vi "FIB profile.vi"(1 "ActiveX Container":refnum<k7>(container), 4 "Capella HV Data Output":T2 {"Column Vac (Torr)" format="%.2e"; "Gun Vac (Torr)" format="%.2e"; "Lens2 Actual (V)" format="%.1f"; "Lens1 Actual (V)" format="%.1f"; "Emission Actual (uA)" format="%.3f"; "Extrator Actual (V)" format="%.1f"; "Tip Lifetime (uAhr)" format="%.2f"; "Lens2 Target (V)" format="%.1f"; "Lens1 Target (V)" format="%.1f"; "SuppI (uA)" format="%.3f"; "Suppressor (V)" format="%.1f"; "Emission Target (uA)" format="%.3f"; "Extrator Target (V)" format="%.1f"; "Accelerator Actual (V)" format="%.1f"; "Accelerator Target (V)" format="%.1f"; "Filament (A)" format="%.2f"}, 5 "HV Data Output":T3 {"Tip Lifetime (hr)" format="%.2f"; "Lens2I (uA)" format="%.3f"; "Lens2 (V)" format="%.1f"; "Lens1I (uA)" format="%.3f"; "Lens1 (V)" format="%.1f"; "SuppI (uA)" format="%.3f"; "Suppressor (V)" format="%.1f"; "Emission (uA)" format="%.3f"; "Extrator (V)" format="%.1f"; "AccI (uA)" format="%.3f"; "Acclerator (V)" format="%.1f"; "Filament (A)" format="%.2f"}, 6 "Parameter Names":string[](array[string])=["Faraday Cup Current", "Specimen Current", "Beam Dump 1 Current", "Beam Dump 2 Current"], 7 "Active logging channels":string="Log/ai0:3", 8 "Scan Para":T5={"X resolution"=500, "Z resolution"=500, "X center"=0.0, "Z center"=0.0, "X size (V)"=10.0, "Z size (V)"=10.0, "Frame line rampdown ratio"=-0.1, "Scan rate (Hz)"=2000000, "Oversampling"=2} {"Frame line rampdown ratio" min=-1.0 max=1.0 step=0.05 format="%.2g"; "Scan rate (Hz)" max=4000000 format="%#.6p"}, 9 "Milling para":T1={"X resolution"=4096, "Z resolution"=125001, "X offset (um)"=0.0, "Z offset (um)"=0.0, "X center (um)"=0.0, "Z center (um)"=0.0, "X size (um)"=250.0, "Z size (um)"=250.0, "UL-Ang"=90.0, "UR-Ang"=90.0, "Line milling time (s)"=5.0, "Z-step (nm)"=2.0, "Lines auto pause"=1, "Auto pause"=FALSE, "Mill from Bottom"=FALSE, "FIB FOV (um)"=500.0, "Auto Profile"=FALSE, "Mill start from Last"=FALSE, "FIB PID on"=FALSE, "FIB PID reset"=TRUE, "FIB PID measured"=0, "FIB PID target"=0.0, "FIB PID target slope"=0.0, "FIB PID P"=0.001, "FIB PID I"=0.01, "FIB PID D"=0.0, "Emission (uA)"=1.36, "Suppressor (V)"=50.0, "Auto reheat"=FALSE} caption="Milling Parameters" {"Suppressor (V)" step=0.1 format="%.1g"; "Emission (uA)" step=0.1 format="%.2g"; "FIB PID measured" items=["Spec.", "B.D. 1", "B.D. 2", "Mill", "Spec. +"]; "FIB PID target slope" min=-1 max=1 step=0.1; "UR-Ang" format="%.2f"; "UL-Ang" format="%.2f"; "Z offset (um)" step=0.02 format="%.3g"; "X offset (um)" step=1 format="%.3g"; "FIB FOV (um)" format="%.3g"; "Line milling time (s)" format="%.1f"; "Z center (um)" format="%#.3g"; "X center (um)" format="%#.3g"}, 10 "Options":T6 {"Scan mode" items=["Raster", "Serpentine"]; "Det" items=["Detector A", "Detector B"]}, 11 "HW Config":T7={"FIB X coil"="FIB/ao0", "FIB Y coil"="FIB/ao1", "Beam blank"="FIB/port0/line0", "Ext Scan"="FIB/port0/line1", "Detector"="FIB/ai1", "Shutter Drive"="PXI1Slot2/ao0"}) -> (0 "error out":errorcluster, 2 "Measurements":dbl[][](graph), 3 "Info & Status":T4={"Actual scan rate"=2000000.0, "X resolution with rampdown"=552, "Actual sample rate"=4000000.0, "Fetch backlog"=664878.0, "Total scan points"=276000, "Frame rate (/s)"=7} {"Fetch backlog" format="%#_6p"; "Actual sample rate" format="%#_6p"; "Actual scan rate" format="%#_4p"})   [LabVIEW 2018]
uses:
  <vilib>/DAQmx/write.llb/DAQmx Write (Digital Wfm 1Chan NSamp).vi
  <vilib>/DAQmx/write.llb/DAQmx Write (Analog 2D DBL NChan NSamp).vi
  <vilib>/DAQmx/read.llb/DAQmx Read (Analog 2D DBL NChan NSamp).vi
  <vilib>/DAQmx/create/channels.llb/DAQmx Create Channel (AI-Voltage-Basic).vi
  <vilib>/Waveform/DWDTOps.llb/DWDT Invert Digital.vi
  <vilib>/DAQmx/create/channels.llb/DAQmx Create Channel (AO-Voltage-Basic).vi
  <vilib>/DAQmx/create/channels.llb/DAQmx Create Channel (DO-Digital Output).vi
  <vilib>/Waveform/DWDTOps.llb/Digital Pattern Generator (Single Value).vi
  <vilib>/Waveform/DWDTOps.llb/DWDT Replace Subset.vi
  <vilib>/DAQmx/configure/timing.llb/DAQmx Timing (Sample Clock).vi
  <vilib>/DAQmx/create/channels.llb/DAQmx Create Channel (CO-Pulse Generation-Frequency).vi
  <vilib>/DAQmx/configure/trigger.llb/DAQmx Start Trigger (Digital Edge).vi
  <vilib>/Waveform/DWDTOps.llb/DWDT Uncompress Digital.vi
  <vilib>/DAQmx/miscellaneous.llb/DAQmx Fill In Error Info.vi
  <vilib>/Utility/file.llb/Write To Spreadsheet File (string).vi
  <resource>/objmgr/daqmx.rc
panel:
  out "Blanking":digitalwaveform(graph)
  in  "COM port":refnum<visa-resource-name>="COM1"
  out "Mill from Bottom":bool
  out "Y scan pattern":dbl[](array[numeric])
  out "AI SampleClk.MaxRate":dbl
  in  "Machine Type":u8(ring) items=["Feiss", "NVision", "Jeiss"]
  out "Ext scan":tag
  out "FIB Y coil":tag="PXI1Slot7/ao1"
  out "FIB X coil":tag="PXI1Slot7/ao0"
  in  "Beam blanked":bool
  out "Beam blank":tag="PXI1Slot7/port0/line0"
  out "Oversampling":u16=2
  out "Frame line rampdown ratio":dbl=0.1
  out "Y end":dbl=1.0
  out "X end":dbl=1.0
  out "Y start":dbl=-1.0
  out "X start":dbl=-1.0
  out "Y resolution":u32=500
  out "X resolution":u32=500
  out "Flip z":bool
  out "Flip x":bool
  out "Scan mode":u16
  in  "stop":bool=TRUE
  # "Direction"
  # "Start\nfrom"
  # "<"
  # "Flip"
  # "Scan coils"
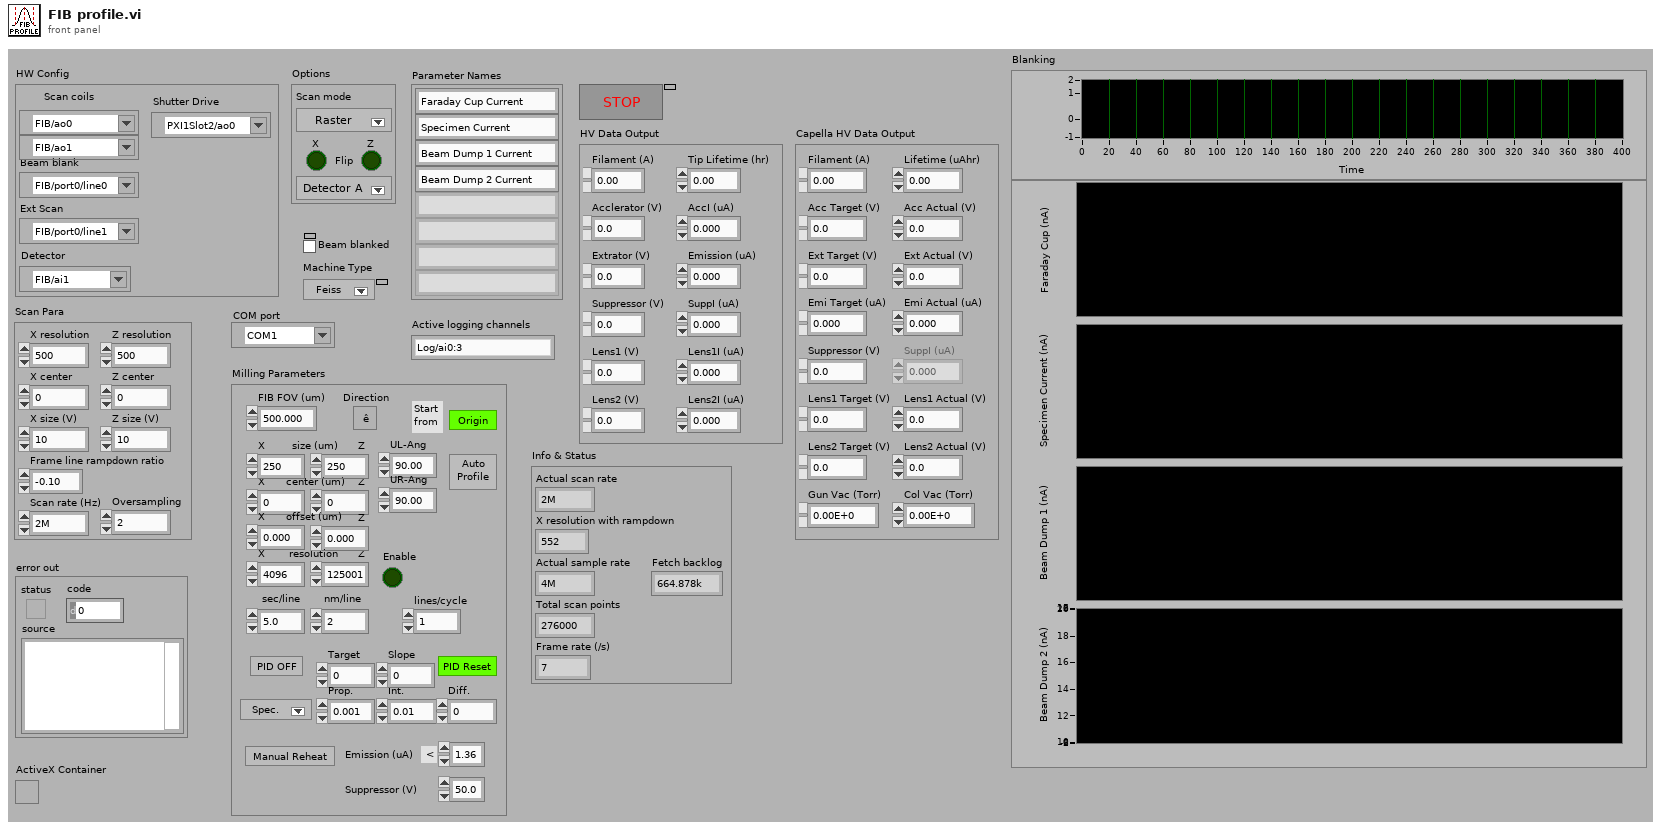
[diagram p1: front panel]
types:
  T1 = cluster{"X resolution":u32, "Z resolution":u32, "X offset (um)":sgl, "Z offset (um)":sgl, "X center (um)":sgl, "Z center (um)":sgl, "X size (um)":sgl, "Z size (um)":sgl, "UL-Ang":sgl, "UR-Ang":sgl, "Line milling time (s)":sgl, "Z-step (nm)":dbl, "Lines auto pause":u16, "Auto pause":bool, "Mill from Bottom":bool, "FIB FOV (um)":sgl, "Auto Profile":bool, "Mill start from Last":bool, "FIB PID on":bool, "FIB PID reset":bool, "FIB PID measured":u8, "FIB PID target":sgl, "FIB PID target slope":sgl, "FIB PID P":sgl, "FIB PID I":sgl, "FIB PID D":sgl, "Emission (uA)":dbl, "Suppressor (V)":sgl, "Auto reheat":bool}
  T2 = cluster{"Filament (A)":sgl, "Accelerator Target (V)":sgl, "Accelerator Actual (V)":sgl, "Extrator Target (V)":sgl, "Extrator Actual (V)":sgl, "Emission Target (uA)":sgl, "Emission Actual (uA)":sgl, "Suppressor (V)":sgl, "SuppI (uA)":sgl, "Lens1 Target (V)":sgl, "Lens1 Actual (V)":sgl, "Lens2 Target (V)":sgl, "Lens2 Actual (V)":sgl, "Gun Vac (Torr)":sgl, "Column Vac (Torr)":sgl, "Tip Lifetime (uAhr)":sgl}
  T3 = cluster{"Filament (A)":sgl, "Acclerator (V)":sgl, "AccI (uA)":sgl, "Extrator (V)":sgl, "Emission (uA)":sgl, "Suppressor (V)":sgl, "SuppI (uA)":sgl, "Lens1 (V)":sgl, "Lens1I (uA)":sgl, "Lens2 (V)":sgl, "Lens2I (uA)":sgl, "Tip Lifetime (hr)":sgl}
  T4 = cluster{"Actual scan rate":dbl, "X resolution with rampdown":i32, "Actual sample rate":dbl, "Fetch backlog":dbl, "Total scan points":i32, "Frame rate (/s)":u32}
  T5 = cluster{"X resolution":u32, "Z resolution":u32, "X center":dbl, "Z center":dbl, "X size (V)":dbl, "Z size (V)":dbl, "Frame line rampdown ratio":dbl, "Scan rate (Hz)":u32, "Oversampling":u16}
  T6 = cluster{"Scan mode":u16, "Flip x":bool, "Flip z":bool, "Det":u16}
  T7 = cluster{"FIB X coil":tag, "FIB Y coil":tag, "Beam blank":tag, "Ext Scan":tag, "Detector":tag, "Shutter Drive":tag}
  T8 = enum16{"SEM", "FIB", "Milling", "SEM + FIB", "Mill + SEM", "SEM Drift Correction", "FIB Drift Correction", "No Beam", "External", "External + SEM"}
  T9 = enum16{"SEM", "FIB", "Mill", "SEM + FIB", "Mill + SEM", "Drift SEM", "Drift FIB", "None", "Ext", "Ext + SEM"}
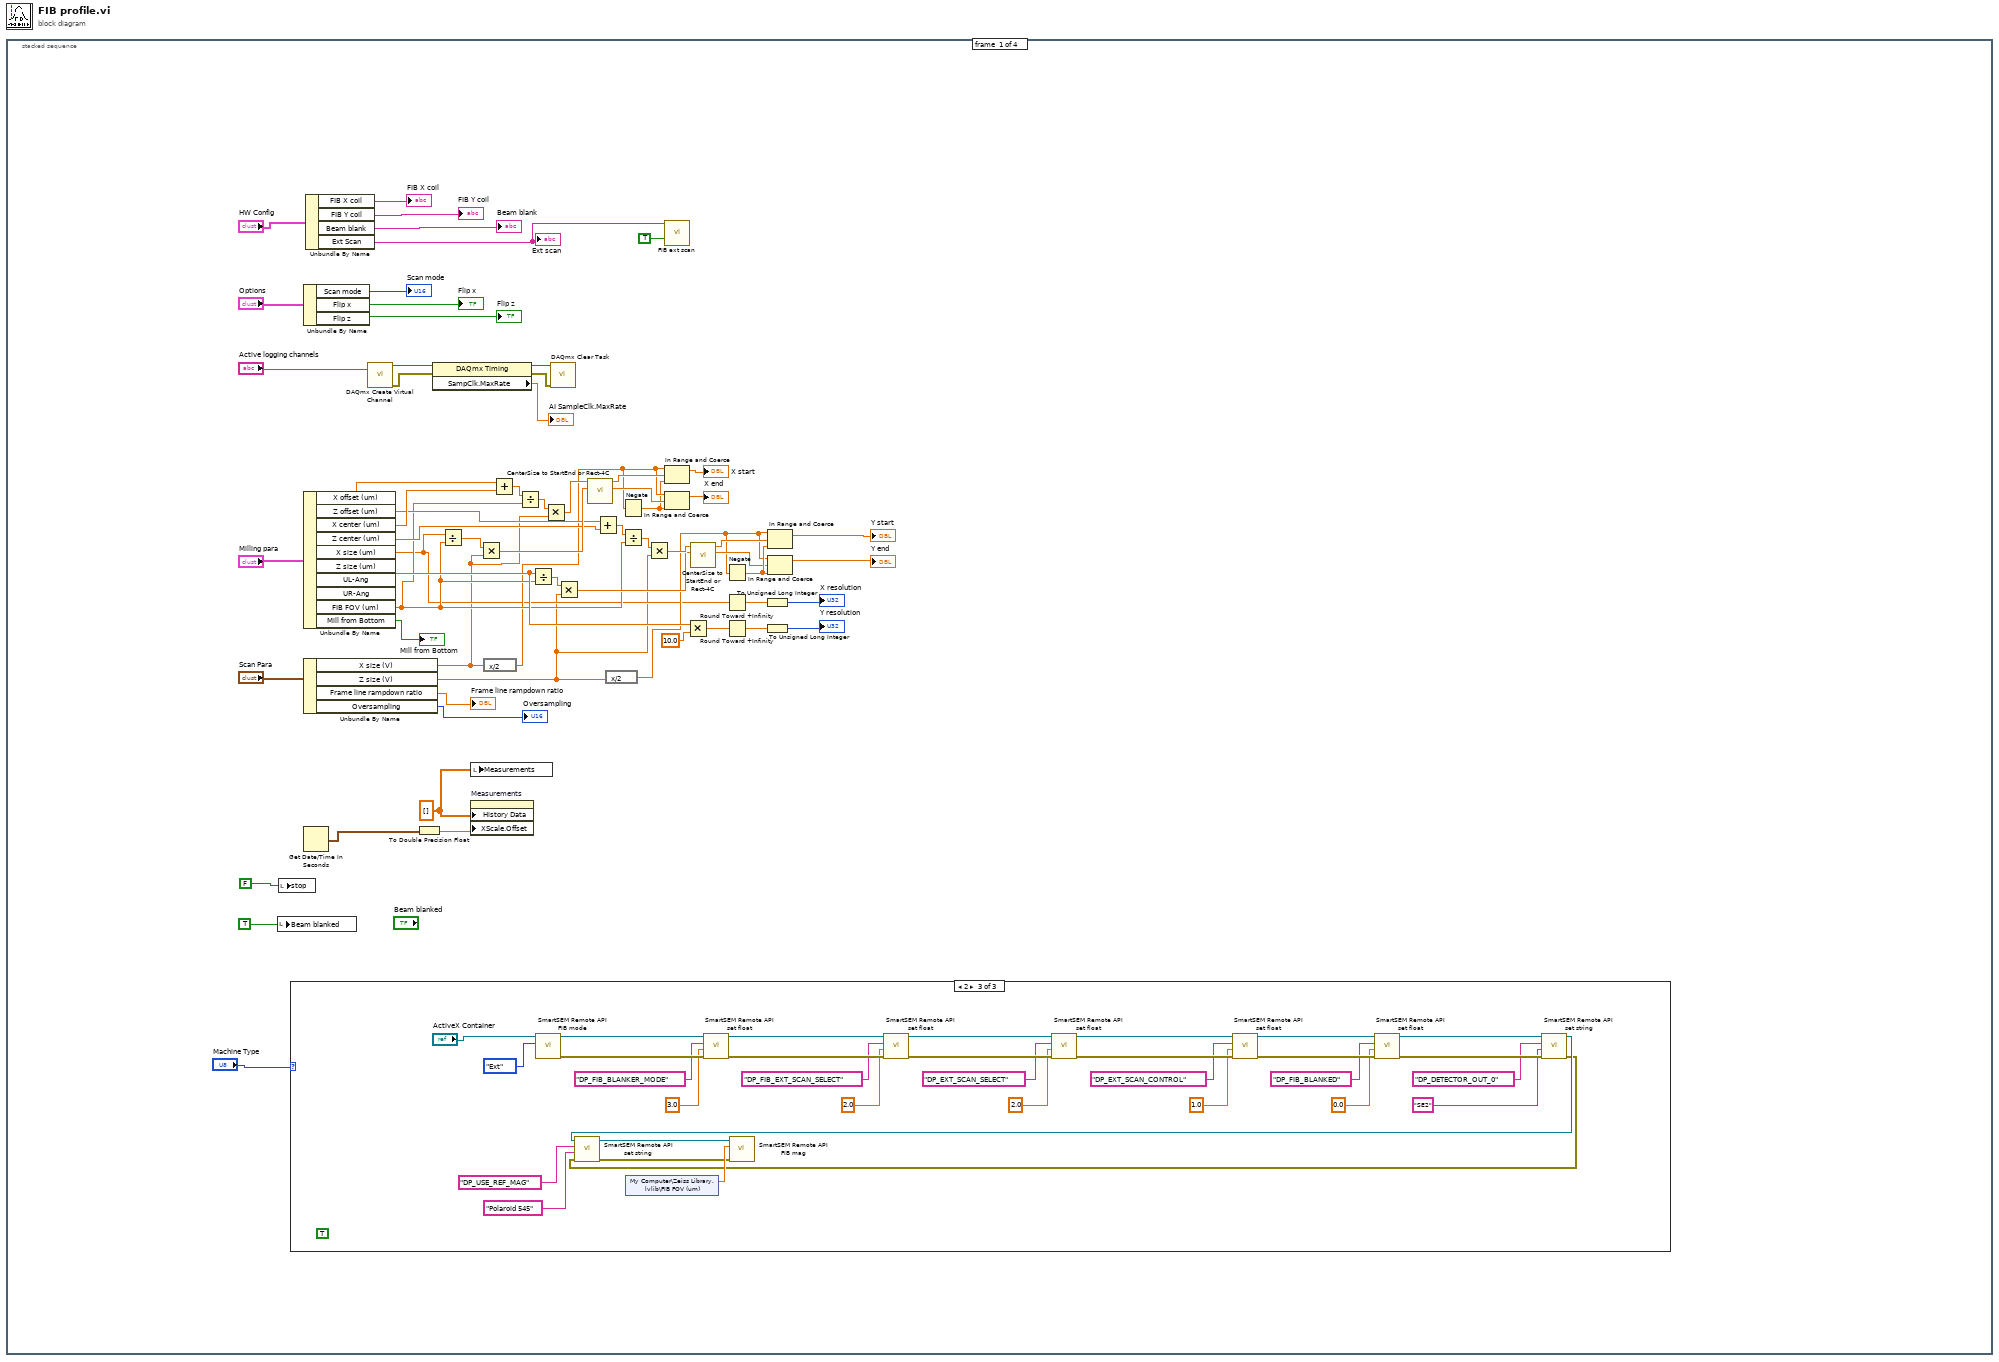
[diagram p0: block diagram]
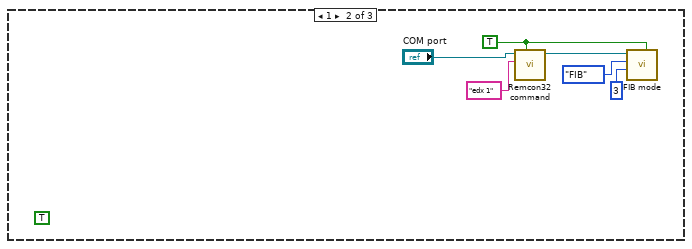
[diagram p3: hidden frame]
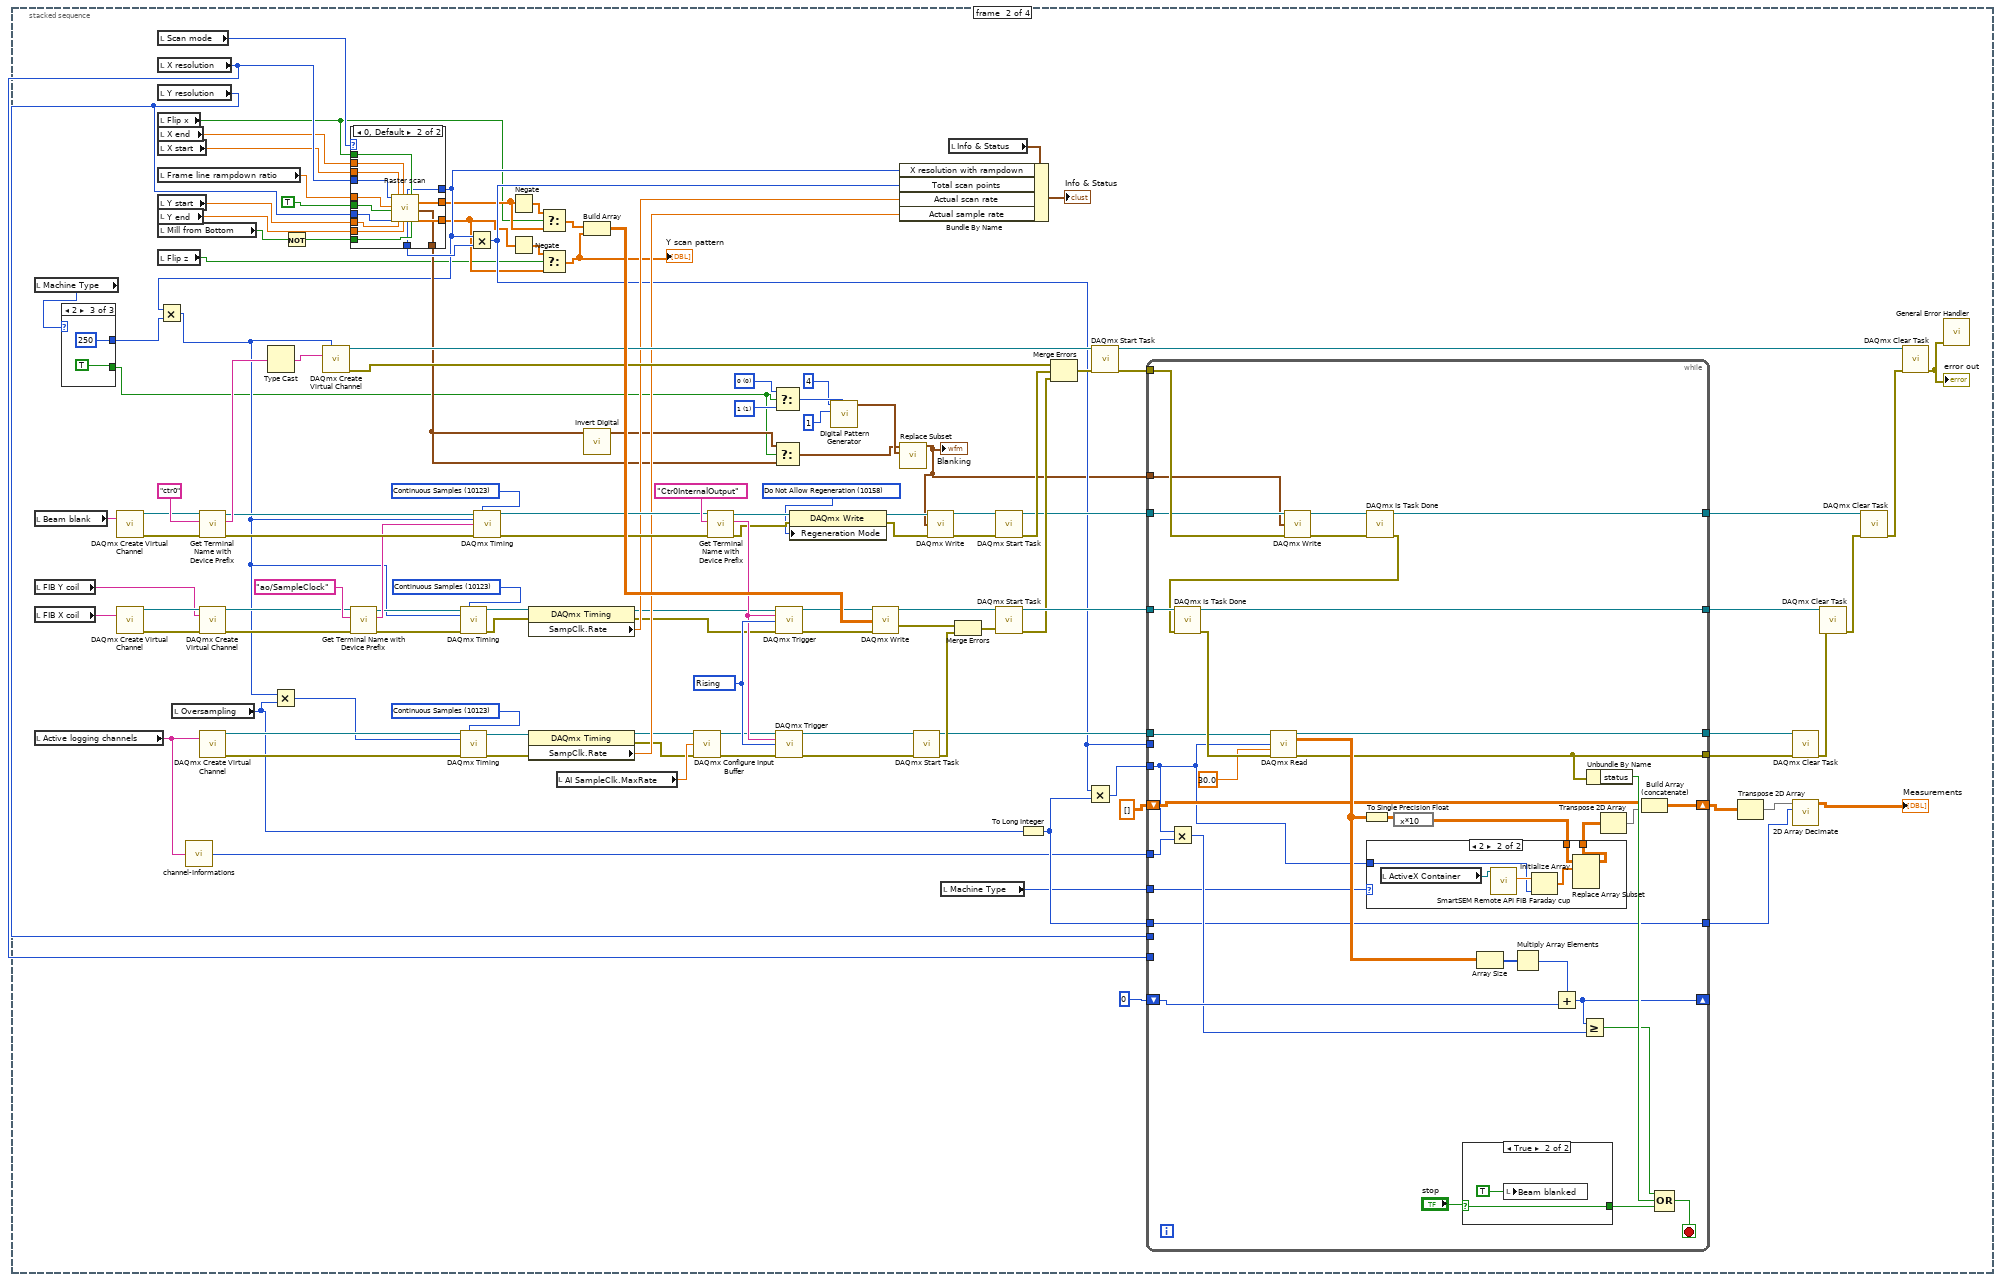
[diagram p4: hidden frame]
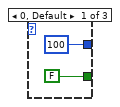
[diagram p5: hidden frame]
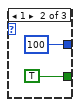
[diagram p6: hidden frame]
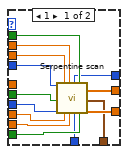
[diagram p7: hidden frame]
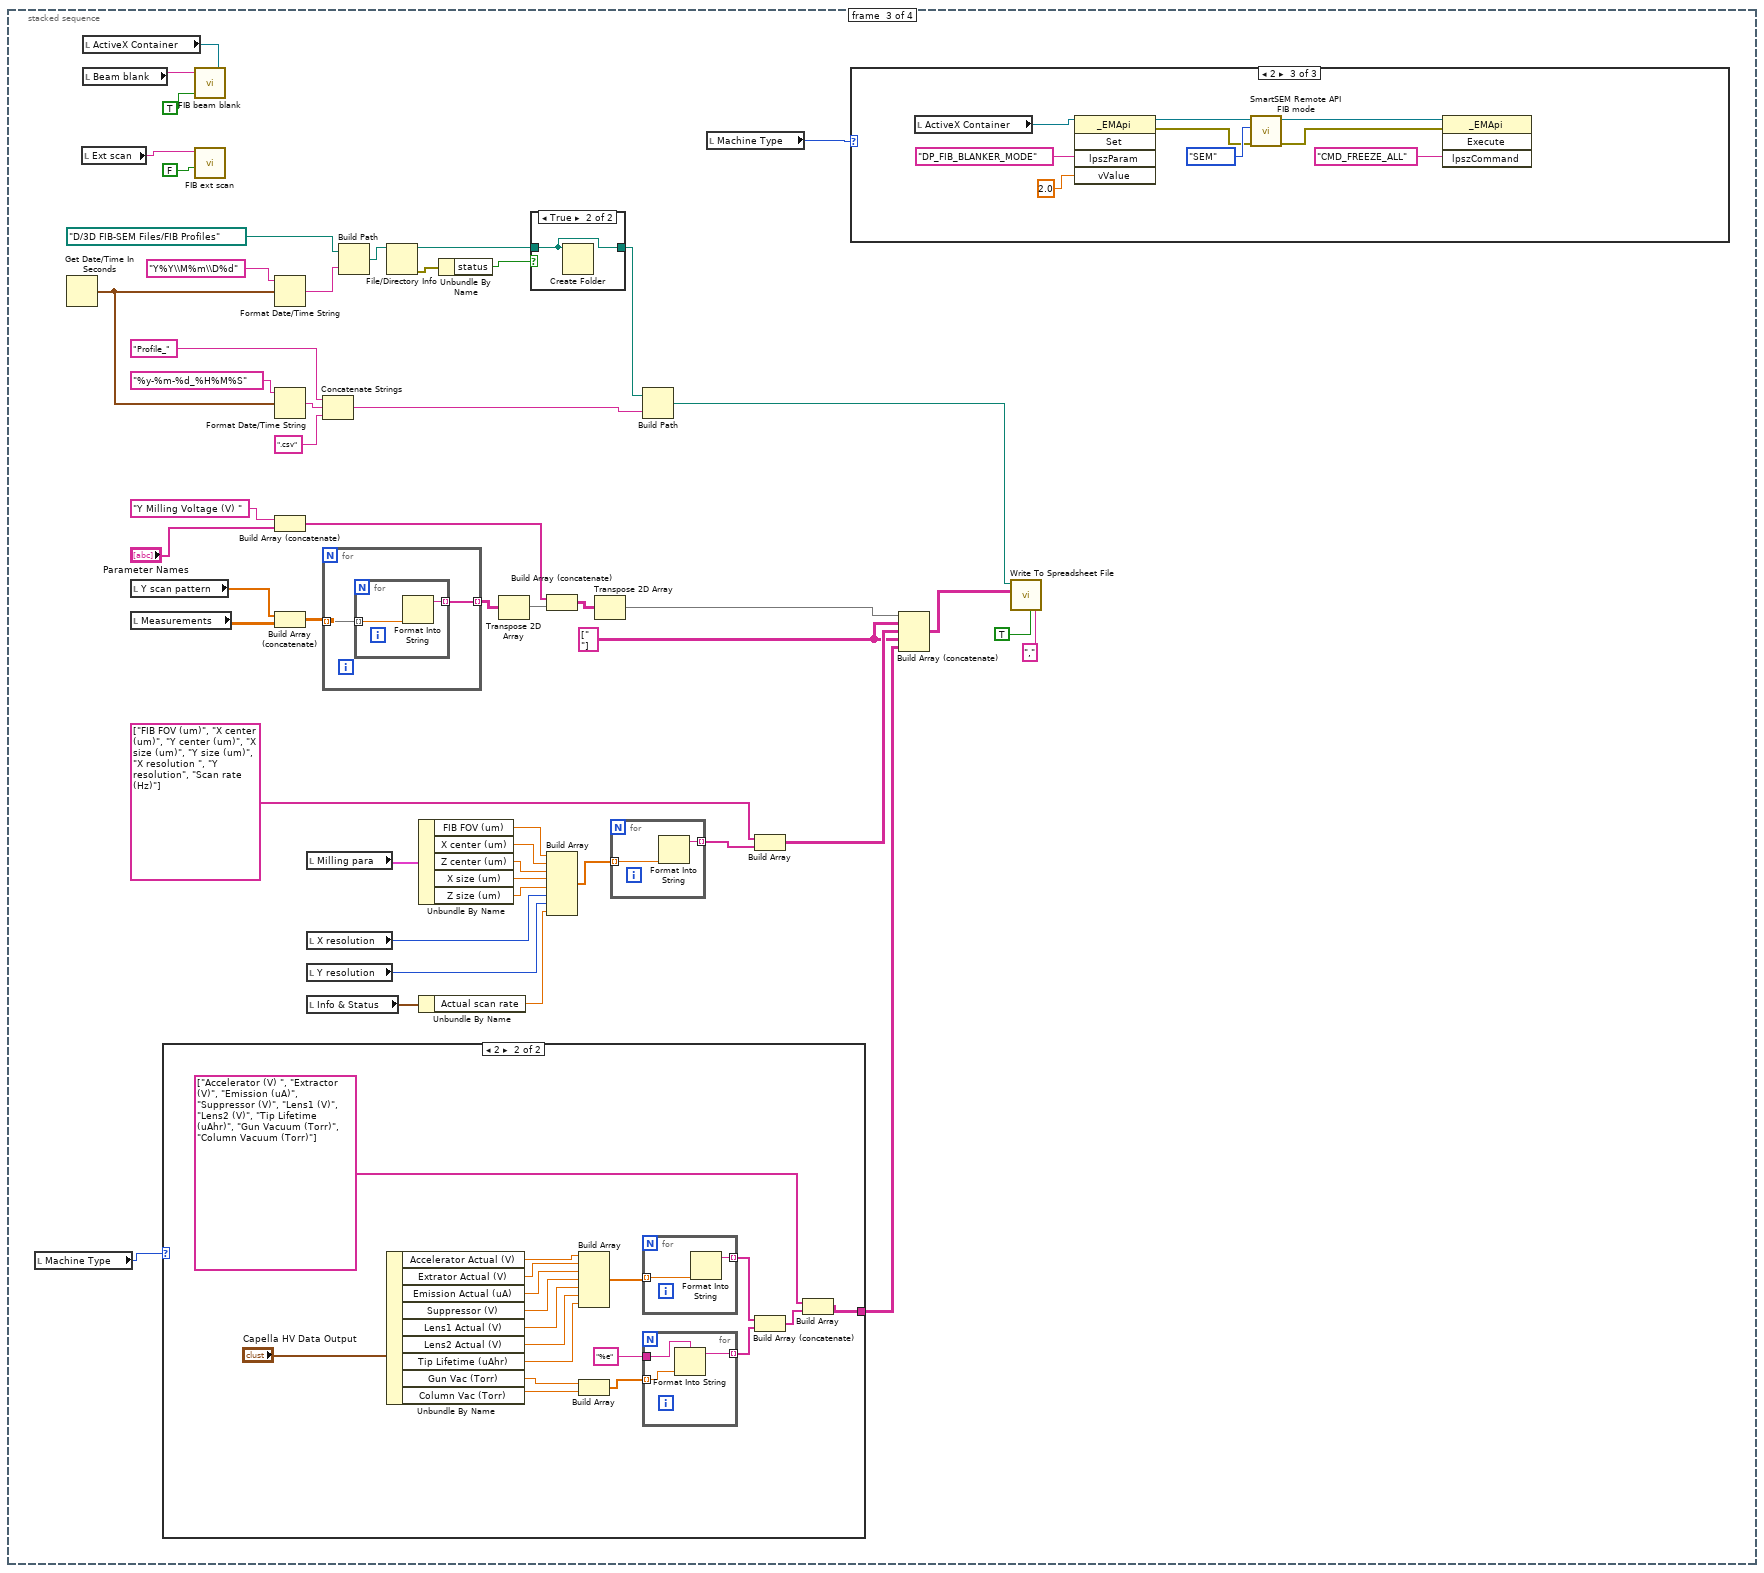
[diagram p10: hidden frame]
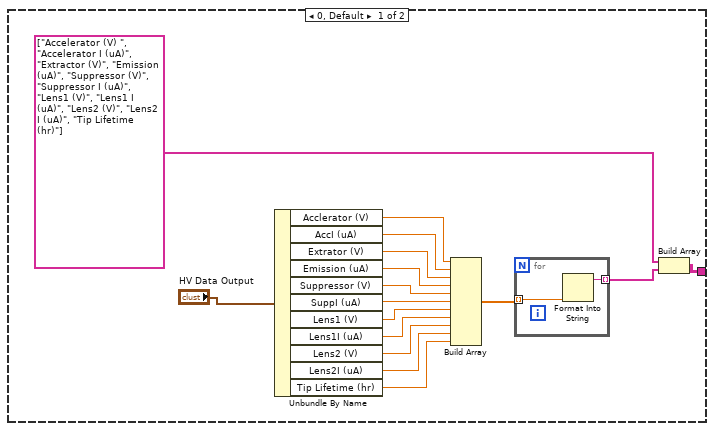
[diagram p11: hidden frame]
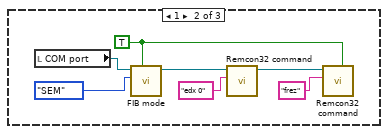
[diagram p13: hidden frame]
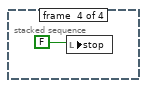
[diagram p15: hidden frame]
diagram:
  n1 = stacked-sequence {
    frame #0 {
      w7 = dbl[][] [] ("History Data")
      n2 = local write "Beam blanked"(TRUE ("Beam blanked")) -> ()
      n3 = local write "stop"(FALSE ("stop")) -> ()
      n4 = case shown="2" "Machine Type" {
        frame 0, Default {
        }
        frame 1 {
          w68 = TRUE ("Close session")
          (unwired) TRUE ("Beam blanked")
          n5 = call "Remcon32 command.vi"("Initialization"=w68, "SEM command"="edx 1", "COM port in"="COM port") -> ("COM port out"=w67:refnum<visa-resource-name>)  [unwired: 5 in, 3 out]
          n6 = call "FIB mode.vi"("Close session"=w68, "Iterations"=u32 3, "FIB mode"=T8."FIB", "COM port in"=w67) -> ()  [unwired: 6 in, 2 out]
        }
        frame 2 {
          (unwired) TRUE ("Beam blanked")
          n7 = call "SmartSEM Remote API FIB mode.vi"("FIB mode"=T9."Ext", "ActiveX Container"="ActiveX Container") -> ("error out"=w100:errorcluster, "reference out"=w101:refnum<k7>)  [unwired: 8 in]
          n8 = shared-variable "My Computer\\Zeiss Library.lvlib\\FIB FOV (um)"() -> (w77:sgl)  [unwired: 1 in, 1 out]
          n9 = call "SmartSEM Remote API set float.vi"("error in"=w100, "vValue"=sgl 3.0, "lpszParam"="DP_FIB_BLANKER_MODE", "ActiveX Container"=w101) -> ("error out"=w96:errorcluster, "reference out"=w97:refnum<k7>)  [unwired: 6 in]
          n10 = call "SmartSEM Remote API set float.vi"("error in"=w96, "vValue"=sgl 2.0, "lpszParam"="DP_FIB_EXT_SCAN_SELECT" ("lpszCommand"), "ActiveX Container"=w97) -> ("error out"=w93:errorcluster, "reference out"=w72:refnum<k7>)  [unwired: 6 in]
          n11 = call "SmartSEM Remote API set float.vi"("vValue"=sgl 2.0, "lpszParam"="DP_EXT_SCAN_SELECT" ("lpszCommand"), "ActiveX Container"=w72) -> ("reference out"=w71:refnum<k7>)  [unwired: 7 in, 1 out]
          n12 = call "SmartSEM Remote API set float.vi"("error in"=w93, "vValue"=sgl 1.0, "lpszParam"="DP_EXT_SCAN_CONTROL" ("lpszCommand"), "ActiveX Container"=w71) -> ("error out"=w89:errorcluster, "reference out"=w90:refnum<k7>)  [unwired: 6 in]
          n13 = call "SmartSEM Remote API set float.vi"("error in"=w89, "vValue"=sgl 0.0, "lpszParam"="DP_FIB_BLANKED", "ActiveX Container"=w90) -> ("error out"=w85:errorcluster, "reference out"=w86:refnum<k7>)  [unwired: 6 in]
          n14 = call "SmartSEM Remote API set string.vi"("error in"=w85, "vValue"="SE2" ("Det A Type"), "lpszParam"="DP_DETECTOR_OUT_0", "ActiveX Container"=w86) -> ("error out"=w73:errorcluster, "reference out"=w74:refnum<k7>)  [unwired: 6 in]
          n15 = call "SmartSEM Remote API set string.vi"("error in"=w73, "vValue"="Polaroid 545" ("lpszParam"), "lpszParam"="DP_USE_REF_MAG", "ActiveX Container"=w74) -> ("error out"=w76:errorcluster, "reference out"=w78:refnum<k7>)  [unwired: 6 in]
          n16 = call "SmartSEM Remote API FIB mag.vi"("error in"=w76, "FIB FOV (um)"=w77, "ActiveX Container"=w78) -> ()  [unwired: 7 in, 2 out]
        }
      }
      n17 = Unbundle By Name("Options") -> ("Scan mode"=→"Scan mode":u16, "Flip x"=→"Flip x":bool, "Flip z"=→"Flip z":bool)
      n18 = Unbundle By Name("Milling para") -> ("X offset (um)"=w52:sgl, "Z offset (um)"=w48:sgl, "X center (um)"=w51:sgl, "Z center (um)"=w47:sgl, "X size (um)"=w14:sgl, "Z size (um)"=w40:sgl, "FIB FOV (um)"=w28:sgl, "Mill from Bottom"=→"Mill from Bottom":bool)  [unwired: 2 out]
      n19 = Unbundle By Name("Scan Para") -> ("X size (V)"=w3:dbl, "Z size (V)"=w4:dbl, "Frame line rampdown ratio"=→"Frame line rampdown ratio":dbl, "Oversampling"=→"Oversampling":u16)
      n20 = Get Date/Time In Seconds() -> (seconds since 1Jan1904=w9:timestamp)
      n21 = Unbundle By Name("HW Config") -> ("FIB X coil"=→"FIB X coil":tag, "FIB Y coil"=→"FIB Y coil":tag, "Beam blank"=→"Beam blank":tag, "Ext Scan"=w56:tag)
      "Ext scan" <- w56
      n22 = call-poly <vilib>:"DAQmx Create Virtual Channel.vi"("physical channels"="Active logging channels") -> ("task out"=w37:refnum<k21>, "error out"=w35:errorcluster)  [unwired: 8 in, 5 out]
      n23 = To Double Precision Float(number=w9) -> (double precision float=w8:dbl)
      n24 = property class="DAQmx Timing"(reference=w37, error in=w35) -> (reference out=w38:refnum<k21>, error out=w36:errorcluster, "SampClk.MaxRate"=→"AI SampleClk.MaxRate":dbl)
      n25 = Divide(x=w14, y=w28) -> (x/y=w53:sgl)
      n26 = local write "Measurements"(w7) -> ()
      n27 = property on="Measurements" class="WFChart (strict)"("History Data"=w7, "XScale.Offset"=w8) -> ()  [unwired: 2 in, 2 out]
      n28 = Multiply(x=w53, y=w3) -> (x*y=w49:dbl)
      n29 = expression code="x/2"(w3) -> (w23:dbl)
      n30 = Add(x=w52, y=w51) -> (x+y=w29:sgl)
      n31 = Divide(x=w29, y=w28) -> (x/y=w30:sgl)
      n32 = Divide(x=w40, y=w28) -> (x/y=w46:sgl)
      n33 = Multiply(x=w30, y=w3) -> (x*y=w50:dbl)
      n34 = call <vilib>:"DAQmx Clear Task.vi"("task in"=w38, "error in"=w36) -> ()  [unwired: 14 out]
      n35 = Multiply(x=w46, y=w4) -> (x*y=w44:dbl)
      n36 = call "CenterSize to StartEnd or Rect-4C.vi"("Size"=w49, "Center"=w50) -> ("End"=w25:dbl, "Start"=w27:dbl)  [unwired: 3 in, 1 out]
      n37 = Add(x=w48, y=w47) -> (x+y=w32:sgl)
      n38 = expression code="x/2"(w4) -> (w16:dbl)
      n39 = Negate(x=w23) -> (-x=w22:dbl)
      n40 = Divide(x=w32, y=w28) -> (x/y=w31:sgl)
      n41 = Multiply(x=w31, y=w4) -> (x*y=w45:dbl)
      n42 = call "FIB ext scan.vi"("Ext on"=TRUE ("data"), "FIB Ext Scan"=w56) -> ()  [unwired: 9 in, 1 out]
      n43 = In Range and Coerce(upper limit=w23, x=w27, lower limit=w22) -> (coerced(x)=→"X start":dbl)  [unwired: 1 out]
      n44 = In Range and Coerce(upper limit=w23, x=w25, lower limit=w22) -> (coerced(x)=→"X end":dbl)  [unwired: 1 out]
      n45 = Multiply(x=w40, y=sgl 10.0) -> (x*y=w15:sgl)
      n46 = call "CenterSize to StartEnd or Rect-4C.vi"("Size"=w44, "Center"=w45) -> ("End"=w17:dbl, "Start"=w18:dbl)  [unwired: 3 in, 1 out]
      n47 = Negate(x=w16) -> (-x=w21:dbl)
      n48 = Round Toward +Infinity(x=w14) -> (ceil(x): smallest int >= x=w13:sgl)
      n49 = Round Toward +Infinity(x=w15) -> (ceil(x): smallest int >= x=w12:sgl)
      n50 = To Unsigned Long Integer(number=w13) -> (unsigned 32bit integer=→"X resolution":u32)
      n51 = To Unsigned Long Integer(number=w12) -> (unsigned 32bit integer=→"Y resolution":u32)
      n52 = In Range and Coerce(upper limit=w16, x=w18, lower limit=w21) -> (coerced(x)=→"Y start":dbl)  [unwired: 1 out]
      n53 = In Range and Coerce(upper limit=w16, x=w17, lower limit=w21) -> (coerced(x)=→"Y end":dbl)  [unwired: 1 out]
    }
    frame #1 {
      w111 = u8 1 items=["0", "1", "Z", "L", "H", "X", "T", "V"] ("value")
      w148 = u8 0 items=["0", "1", "Z", "L", "H", "X", "T", "V"] ("value")
      w157 = 10158 items=["Allow Regeneration"=10097, "Do Not Allow Regeneration"=10158] ("RegenMode")
      w181 = 10123 items=["Finite Samples"=10178, "Continuous Samples"=10123] ("sample mode")
      w169 = 10280 items=["Rising"=10280, "Falling"=10171] ("edge")
      w206 = 10123 items=["Finite Samples"=10178, "Continuous Samples"=10123, "Hardware Timed Single Point"=12522] ("sample mode")
      w210 = 10123 items=["Finite Samples"=10178, "Continuous Samples"=10123, "Hardware Timed Single Point"=12522] ("sample mode")
      n54 = local read "Machine Type"() -> (w105:u8)
      n55 = local read "Beam blank"() -> (w153:tag)
      n56 = local read "FIB Y coil"() -> (w211:tag)
      n57 = local read "FIB X coil"() -> (w212:tag)
      n58 = local read "Active logging channels"() -> (w140:string)
      n59 = case shown="2" w105 {
        tunnel: [u32 100 ("x") u32 100 ("x") u32 250 ("x")] -> w104
        tunnel: [FALSE ("Flip x") TRUE ("Flip x") TRUE ("Flip x")] -> w103
        frame 0, Default {
        }
        frame 1 {
        }
        frame 2 {
        }
      }
      n60 = call-poly <vilib>:"DAQmx Create Virtual Channel.vi"("lines"=w153) -> ("task out"=w188:refnum<k21>, "error out"=w190:errorcluster)  [unwired: 6 in, 7 out]
      n61 = call-poly <vilib>:"DAQmx Create Virtual Channel.vi"("physical channels"=w212) -> ("task out"=w214:refnum<k21>, "error out"=w213:errorcluster)  [unwired: 8 in, 5 out]
      n62 = local read "Scan mode"() -> (w226:u16)
      n63 = local read "X resolution"() -> (w225:u32)
      n64 = local read "Y resolution"() -> (w224:u32)
      n65 = local read "Flip x"() -> (w113:bool)
      n66 = local read "X end"() -> (w217:dbl)
      n67 = local read "X start"() -> (w218:dbl)
      n68 = local read "Frame line rampdown ratio"() -> (w223:dbl)
      n69 = local read "Y start"() -> (w216:dbl)
      n70 = local read "Y end"() -> (w215:dbl)
      n71 = local read "Mill from Bottom"() -> (w122:bool)
      n72 = local read "Flip z"() -> (w118:bool)
      n73 = local read "Oversampling"() -> (w162:u16)
      n74 = call "channel-Informations.vi"("Channel Name"=w140) -> ("No. of channels:"=w139:i32)  [unwired: 2 out]
      n75 = call "Get Terminal Name with Device Prefix.vi"("error in"=w190, "Local Terminal Name"="ctr0", "task/channels in"=w188) -> ("error out"=w191:errorcluster, "Terminal Name with Device Prefix"=w193:tag, "task out"=w189:refnum<k21>)  [unwired: 6 in]
      n76 = call-poly <vilib>:"DAQmx Create Virtual Channel.vi"("task in"=w214, "physical channels"=w211, "error in"=w213) -> ("task out"=w145:refnum<k21>, "error out"=w144:errorcluster)  [unwired: 6 in, 5 out]
      n77 = call-poly <vilib>:"DAQmx Create Virtual Channel.vi"("physical channels"=w140) -> ("task out"=w208:refnum<k21>, "error out"=w207:errorcluster)  [unwired: 8 in, 5 out]
      n78 = Type Cast(x=w193) -> (*(type *) &x=w194:string)  [unwired: 1 in]
      n79 = Not(x=w122) -> (.not. x?=w112:bool)
      n80 = case shown="0, Default" w226 {
        tunnel: w223 -> [_ w260]
        tunnel: w113 -> [w243 w263]
        tunnel: w224 -> [w246 w258]
        tunnel: w225 -> [w248 w261]
        tunnel: w112 -> [w240 w262]
        tunnel: [w239 w257] -> w129
        tunnel: [w238 w256] -> w220
        tunnel: TRUE ("Flip x") -> [w247 w259]
        tunnel: w218 -> [w245 w255]
        tunnel: w217 -> [w244 w254]
        tunnel: w216 -> [w242 w253]
        tunnel: w215 -> [w241 w252]
        tunnel: [w237 w251] -> w114
        tunnel: [w236 w250] -> w120
        tunnel: [w235 w249] -> w146
        frame 1 {
          n81 = call "Serpentine scan.vi"("X resolution"=w248, "Scan pattern?"=w247, "Y resolution"=w246, "X start"=w245, "Y start"=w242, "X end"=w244, "Y end"=w241, "Flip x"=w243, "Flip y"=w240) -> ("X resolution with rampdown"=w239:i32, "Y resolution"=w238:i32, "X scan pattern"=w237:dbl[], "Blanking pattern"=w235:digitalwaveform, "Y scan pattern"=w236:dbl[])  [unwired: 3 in, 3 out]
        }
        frame 0, Default {
          n82 = call "Raster scan.vi"("X resolution"=w261, "Frame line rampdown ratio"=w260, "Scan pattern?"=w259, "Y resolution"=w258, "X start"=w255, "Y start"=w253, "X end"=w254, "Y end"=w252, "Flip x"=w263, "Flip y"=w262) -> ("X resolution with rampdown"=w257:i32, "Y resolution"=w256:i32, "X scan pattern"=w251:dbl[], "Blanking pattern"=w249:digitalwaveform, "Y scan pattern"=w250:dbl[])  [unwired: 2 in, 3 out]
        }
      }
      n83 = Multiply(x=w129, y=w104) -> (x*y=w130:u32)
      n84 = Multiply(x=w130, y=w162) -> (x*y=w163:u32)
      n85 = call-poly <vilib>:"DAQmx Create Virtual Channel.vi"("frequency"=w130, "counter"=w194) -> ("task out"=w184:refnum<k21>, "error out"=w186:errorcluster)  [unwired: 7 in, 5 out]
      n86 = call "Get Terminal Name with Device Prefix.vi"("error in"=w144, "Local Terminal Name"="ao/SampleClock", "task/channels in"=w145) -> ("error out"=w164:errorcluster, "Terminal Name with Device Prefix"=w177:tag, "task out"=w165:refnum<k21>)  [unwired: 6 in]
      n87 = call-poly <vilib>:"DAQmx Timing.vi"("task/channels in"=w165, "sample mode"=w210, "rate"=w130, "error in"=w164) -> ("task out"=w167:refnum<k21>, "error out"=w166:errorcluster)  [unwired: 3 in, 7 out]
      n88 = call-poly <vilib>:"DAQmx Timing.vi"("task/channels in"=w208, "sample mode"=w206, "rate"=w163, "error in"=w207) -> ("task out"=w205:refnum<k21>, "error out"=w204:errorcluster)  [unwired: 3 in, 7 out]
      n89 = Multiply(x=w129, y=w220) -> (x*y=w128:i32)
      n90 = call-poly <vilib>:"DAQmx Timing.vi"("task/channels in"=w189, "sample mode"=w181, "rate"=w130, "source"=w177, "error in"=w191) -> ("task out"=w180:refnum<k21>, "error out"=w179:errorcluster)  [unwired: 2 in, 7 out]
      n91 = Negate(x=w114) -> (-x=w116:dbl[])
      n92 = Negate(x=w120) -> (-x=w121:dbl[])
      n93 = property class="DAQmx Timing"(reference=w167, error in=w166) -> (reference out=w150:refnum<k21>, error out=w149:errorcluster, "SampClk.Rate"=w152:dbl)
      n94 = property class="DAQmx Timing"(reference=w205, error in=w204) -> (reference out=w136:refnum<k21>, error out=w135:errorcluster, "SampClk.Rate"=w151:dbl)
      n95 = Select(t=w116, s=w113, f=w114) -> (s? t:f=w115:dbl[])
      n96 = Select(t=w121, s=w118, f=w120) -> (s? t:f=w119:dbl[])
      "Y scan pattern" <- w119
      n97 = local read "AI SampleClk.MaxRate"() -> (w138:dbl)
      n98 = Build Array(w115, w119) -> (w202:dbl[][])
      n99 = call-poly <vilib>:"Invert Digital.vi"("digital waveform"=w146) -> ("inverted waveform"=w147:digitalwaveform)  [unwired: 9 in, 1 out]
      n100 = call <vilib>:"DAQmx Configure Input Buffer.vi"("task/channels in"=w136, "buffer size (in samples per channel)"=w138, "error in"=w135) -> ("task out"=w137:refnum<k21>, "error out"=w134:errorcluster)  [unwired: 11 in]
      n101 = call "Get Terminal Name with Device Prefix.vi"("error in"=w179, "Local Terminal Name"="Ctr0InternalOutput" ("terminal"), "task/channels in"=w180) -> ("error out"=w159:errorcluster, "Terminal Name with Device Prefix"=w168:tag, "task out"=w161:refnum<k21>)  [unwired: 1 in, 5 out]
      n102 = Select(t=w148, s=w103, f=w111) -> (s? t:f=w110:u8)
      n103 = Select(t=w147, s=w103, f=w146) -> (s? t:f=w107:digitalwaveform)
      n104 = call-poly <vilib>:"DAQmx Trigger.vi"("task/channels in"=w150, "source"=w168, "edge"=w169, "error in"=w149) -> ("task out"=w170:refnum<k21>, "error out"=w171:errorcluster)  [unwired: 10 out]
      n105 = call-poly <vilib>:"DAQmx Trigger.vi"("task/channels in"=w137, "source"=w168, "edge"=w169, "error in"=w134) -> ("task out"=w141:refnum<k21>, "error out"=w203:errorcluster)  [unwired: 10 out]
      n106 = property class="DAQmx Write"(reference=w161, error in=w159, "Regeneration Mode"=w157) -> (reference out=w160:refnum<k21>, error out=w158:errorcluster)
      n107 = call-poly <vilib>:"Digital Pattern Generator.vi"("value"=w110, "number of signals"=u32 1, "number of samples"=u32 4) -> ("digital waveform"=w108:digitalwaveform)  [unwired: 2 in, 6 out]
      n108 = call-poly <vilib>:"DAQmx Write.vi"("task/channels in"=w170, "data"=w202, "error in"=w171) -> ("task out"=w201:refnum<k21>, "error out"=w199:errorcluster)  [unwired: 1 in, 10 out]
      n109 = call-poly <vilib>:"Replace Subset.vi"("new digital waveform"=w108, "digital waveform in"=w107) -> ("digital waveform out"=w106:digitalwaveform)  [unwired: 7 in, 2 out]
      "Blanking" <- w106
      n110 = call <vilib>:"DAQmx Start Task.vi"("task/channels in"=w141, "error in"=w203) -> ("task out"=w131:refnum<k21>, "error out"=w198:errorcluster)  [unwired: 12 out]
      n111 = call-poly <vilib>:"DAQmx Write.vi"("task/channels in"=w160, "data"=w106, "error in"=w158) -> ("task out"=w183:refnum<k21>, "error out"=w178:errorcluster)  [unwired: 2 in, 9 out]
      n112 = local read "Machine Type"() -> (w117:u8)
      n113 = local read "Info & Status"() -> (w222:T4)
      n114 = Bundle By Name(cluster=w222, "X resolution with rampdown"=w129, "Total scan points"=w128, "Actual scan rate"=w152, "Actual sample rate"=w151) -> (→"Info & Status":T4)
      n115 = Merge Errors(w199, w198) -> (w200:errorcluster)
      n116 = call <vilib>:"DAQmx Start Task.vi"("task/channels in"=w183, "error in"=w178) -> ("task out"=w174:refnum<k21>, "error out"=w185:errorcluster)  [unwired: 12 out]
      n117 = call <vilib>:"DAQmx Start Task.vi"("task/channels in"=w201, "error in"=w200) -> ("task out"=w197:refnum<k21>, "error out"=w176:errorcluster)  [unwired: 12 out]
      n118 = To Long Integer(number=w162) -> (32bit integer=w228:i32)
      n119 = Merge Errors(w186, w185, w176) -> (w187:errorcluster)
      n120 = Multiply(x=w128, y=w228) -> (x*y=w227:i32)
      n121 = call <vilib>:"DAQmx Start Task.vi"("task/channels in"=w184, "error in"=w187) -> ("task out"=w173:refnum<k21>, "error out"=w175:errorcluster)  [unwired: 12 out]
      n122 = while {
        tunnel: w228 -> [w269]
        tunnel: w224 -> [_]
        tunnel: w225 -> [_]
        tunnel: w227 -> [w266]
        tunnel: w131 -> [w281]
        tunnel: w197 -> [w295]
        tunnel: [w274] -> w132
        tunnel: [w275] -> w133
        tunnel: [w294] -> w196
        tunnel: w175 -> [w289]
        tunnel: w174 -> [w288]
        tunnel: [w291] -> w172
        tunnel: w106 -> [w264]
        shift-right: [w285] -> _
        shift-left: 0 -> [w286]
        tunnel: w139 -> [w280]
        tunnel: w128 -> [_]
        shift-right: [w272] -> w127
        shift-left: sgl[][] [] -> [w270]
        tunnel: [w269] -> w123
        tunnel: w117 -> [w265]
        stop <- w298 stop-if-true
        n123 = Multiply(x=w266, y=w280) -> (x*y=w276:i32)
        n124 = call-poly <vilib>:"DAQmx Write.vi"("task/channels in"=w288, "data"=w264, "error in"=w289) -> ("task out"=w287:refnum<k21>, "error out"=w290:errorcluster)  [unwired: 2 in, 9 out]
        n125 = call <vilib>:"DAQmx Is Task Done.vi"("task/channels in"=w287, "error in"=w290) -> ("task out"=w291:refnum<k21>, "error out"=w292:errorcluster)  [unwired: 2 in, 10 out]
        n126 = call <vilib>:"DAQmx Is Task Done.vi"("task/channels in"=w295, "error in"=w292) -> ("task out"=w294:refnum<k21>, "error out"=w282:errorcluster)  [unwired: 2 in, 10 out]
        n127 = call-poly <vilib>:"DAQmx Read.vi"("task/channels in"=w281, "number of samples per channel"=w266, "timeout"=30.0, "error in"=w282) -> ("task out"=w275:refnum<k21>, "data"=w279:dbl[][], "error out"=w274:errorcluster)  [unwired: 9 out]
        n128 = To Single Precision Float(number=w279) -> (single precision float=w283:sgl[][])
        n129 = expression code="x*10"(w283) -> (w268:sgl[][])
        n130 = case shown="2" w265 {
          tunnel: w268 -> [w299 w303]
          tunnel: w266 -> [_ w302]
          tunnel: [w299 w301] -> w267
          frame 0, Default {
          }
          frame 2 {
            n131 = local read "ActiveX Container"() -> (w300:refnum<k7>)
            n132 = call "SmartSEM Remote API FIB Faraday cup.vi"("ActiveX Container"=w300) -> ("FIB Faraday Cup (nA)"=w304:sgl)  [unwired: 8 in, 2 out]
            n133 = Initialize Array(w304, w302) -> (w305:sgl[])
            n134 = Replace Array Subset(array=w303, new element=w305) -> (w301:sgl[][])  [unwired: 2 in]
          }
        }
        n135 = case shown="True" "stop" {
          selector: "stop" -> [w306 w308]
          tunnel: [w306 w308] -> w296
          frame False {
          }
          frame True {
            n136 = local write "Beam blanked"(TRUE ("Beam blanked")) -> ()
          }
        }
        n137 = Array Size(array=w279) -> (size(s)=w278:i32[])
        n138 = Multiply Array Elements(1:w278) -> (0:w277:i32)
        n139 = Add(x=w277, y=w286) -> (x+y=w285:i32)
        n140 = Greater Or Equal?(x=w285, y=w276) -> (x >= y?=w284:bool)
        n141 = Unbundle By Name(w274) -> ("status"=w293:bool)
        n142 = Transpose 2D Array(2D array=w267) -> (transposed array=w271:sgl[][])
        n143 = Build Array (concatenate)(w270, w271) -> (w272:sgl[][])
        n144 = Compound Arithmetic op=OR(w284, w293, w296) -> (w298:bool)
      }
      n145 = Transpose 2D Array(2D array=w127) -> (transposed array=w125:sgl[][])
      n146 = call <vilib>:"DAQmx Clear Task.vi"("task in"=w133, "error in"=w132) -> ("error out"=w195:errorcluster)  [unwired: 13 out]
      n147 = call "2D Array Decimate.vi"("x decimating factor"=w123, "Input 2D Array"=w125) -> ("output array"=→"Measurements":dbl[][])  [unwired: 7 in, 2 out]
      n148 = call <vilib>:"DAQmx Clear Task.vi"("task in"=w196, "error in"=w195) -> ("error out"=w155:errorcluster)  [unwired: 13 out]
      n149 = call <vilib>:"DAQmx Clear Task.vi"("task in"=w172, "error in"=w155) -> ("error out"=w154:errorcluster)  [unwired: 13 out]
      n150 = call <vilib>:"DAQmx Clear Task.vi"("task in"=w173, "error in"=w154) -> ("error out"=w142:errorcluster)  [unwired: 13 out]
      "error out" <- w142
      n151 = call <vilib>:"General Error Handler.vi"("error in (no error)"=w142) -> ()  [unwired: 10 in, 5 out]
    }
    frame #2 {
      w313 = string[][] [[" "]] ("array")
      n152 = local read "Machine Type"() -> (w310:u8)
      n153 = Get Date/Time In Seconds() -> (seconds since 1Jan1904=w348:timestamp)
      n154 = local read "Ext scan"() -> (w357:tag)
      n155 = local read "ActiveX Container"() -> (w309:refnum<k7>)
      n156 = local read "Beam blank"() -> (w358:tag)
      n157 = local read "Y scan pattern"() -> (w340:dbl[])
      n158 = local read "Measurements"() -> (w341:dbl[][])
      n159 = case shown="2" w310 {
        tunnel: [w360 w381] -> w312
        frame 0, Default {
          n160 = Unbundle By Name("HV Data Output") -> ("Acclerator (V)"=w374:sgl, "AccI (uA)"=w373:sgl, "Extrator (V)"=w372:sgl, "Emission (uA)"=w371:sgl, "Suppressor (V)"=w370:sgl, "SuppI (uA)"=w369:sgl, "Lens1 (V)"=w368:sgl, "Lens1I (uA)"=w367:sgl, "Lens2 (V)"=w366:sgl, "Lens2I (uA)"=w365:sgl, "Tip Lifetime (hr)"=w364:sgl)
          n161 = Build Array(w374, w373, w372, w371, w370, w369, w368, w367, w366, w365, w364) -> (w363:sgl[])
          n162 = for {
            tunnel: w363 -> [w377] mode=indexing
            tunnel: [w376] -> w362 mode=indexing
            n163 = Format Into String(w377) -> (resulting string=w376:string)  [unwired: 3 in, 1 out]
          }
          n164 = Build Array(string[] ["Accelerator (V) ", "Accelerator I (uA)", "Extractor (V)", "Emission (uA)", "Suppressor (V)", "Suppressor I (uA)", "Lens1 (V)", "Lens1 I (uA)", "Lens2 (V)", "Lens2 I (uA)", "Tip Lifetime (hr)"] ("Parameter Names"), w362) -> (w360:string[][])
        }
        frame 2 {
          n165 = Unbundle By Name("Capella HV Data Output") -> ("Accelerator Actual (V)"=w395:sgl, "Extrator Actual (V)"=w394:sgl, "Emission Actual (uA)"=w393:sgl, "Suppressor (V)"=w392:sgl, "Lens1 Actual (V)"=w391:sgl, "Lens2 Actual (V)"=w390:sgl, "Tip Lifetime (uAhr)"=w386:sgl, "Gun Vac (Torr)"=w383:sgl, "Column Vac (Torr)"=w382:sgl)
          n166 = Build Array(w395, w394, w393, w392, w391, w390, w386) -> (w389:sgl[])
          n167 = Build Array(w383, w382) -> (w385:sgl[])
          n168 = for {
            tunnel: w389 -> [w400] mode=indexing
            tunnel: [w399] -> w379 mode=indexing
            n169 = Format Into String(w400) -> (resulting string=w399:string)  [unwired: 3 in, 1 out]
          }
          n170 = for {
            tunnel: w385 -> [w398] mode=indexing
            tunnel: [w397] -> w378 mode=indexing
            tunnel: "%e" ("format string") -> [w396]
            n171 = Format Into String(format string=w396, w398) -> (resulting string=w397:string)  [unwired: 2 in, 1 out]
          }
          n172 = Build Array (concatenate)(w379, w378) -> (w380:string[])
          n173 = Build Array(string[] ["Accelerator (V) ", "Extractor (V)", "Emission (uA)", "Suppressor (V)", "Lens1 (V)", "Lens2 (V)", "Tip Lifetime (uAhr)", "Gun Vacuum (Torr)", "Column Vacuum (Torr)"] ("Parameter Names"), w380) -> (w381:string[][])
        }
      }
      n174 = call "FIB beam blank.vi"("ActiveX Container"=w309, "Beam blanked"=TRUE, "lines"=w358) -> ()  [unwired: 2 in, 1 out]
      n175 = call "FIB ext scan.vi"("Ext on"=FALSE ("data"), "FIB Ext Scan"=w357) -> ()  [unwired: 9 in, 1 out]
      n176 = Format Date/Time String(time format string (%c)="Y%Y\\M%m\\D%d", seconds (now)=w348) -> (date/time string=w355:string)  [unwired: 1 out]
      n177 = Format Date/Time String(time format string (%c)="%y-%m-%d_%H%M%S", seconds (now)=w348) -> (date/time string=w347:string)  [unwired: 1 out]
      n178 = Build Array (concatenate)("Y Milling Voltage (V) " ("string"), "Parameter Names") -> (w332:string[])
      n179 = Build Array (concatenate)(w340, w341) -> (w339:dbl[][])
      n180 = local read "Milling para"() -> (w327:T1)
      n181 = local read "X resolution"() -> (w316:u32)
      n182 = local read "Y resolution"() -> (w315:u32)
      n183 = local read "Info & Status"() -> (w317:T4)
      n184 = Concatenate Strings("Profile_" ("string"), w347, ".csv" ("string")) -> (w345:string)
      n185 = for {
        tunnel: w339 -> [w420] mode=indexing
        tunnel: [w419] -> w334 mode=indexing
        n186 = for {
          tunnel: w420 -> [w422] mode=indexing
          tunnel: [w421] -> w419 mode=indexing
          n187 = Format Into String(w422) -> (resulting string=w421:string)  [unwired: 3 in, 1 out]
        }
      }
      n188 = Build Path(base path=path "D:/3D FIB-SEM Files/FIB Profiles" ("path"), name or relative path=w355) -> (appended path=w344:path)
      n189 = File/Directory Info(path=w344) -> (path out=w351:path, error out=w353:errorcluster)  [unwired: 1 in, 5 out]
      n190 = Unbundle By Name(w327) -> ("FIB FOV (um)"=w326:sgl, "X center (um)"=w325:sgl, "Z center (um)"=w324:sgl, "X size (um)"=w323:sgl, "Z size (um)"=w322:sgl)
      n191 = Unbundle By Name(w317) -> ("Actual scan rate"=w314:dbl)
      n192 = Unbundle By Name(w353) -> ("status"=w352:bool)
      n193 = Transpose 2D Array(2D array=w334) -> (transposed array=w333:string[][])
      n194 = case shown="True" w352 {
        tunnel: w351 -> [w423 w424]
        tunnel: [w423 w424] -> w343
        frame False {
        }
        frame True {
          n195 = Create Folder(path (use dialog)=w424) -> ()  [unwired: 1 in, 4 out]
        }
      }
      n196 = Build Array (concatenate)(w332, w333) -> (w329:string[][])
      n197 = Build Array(w326, w325, w324, w323, w322, w316, w315, w314) -> (w321:dbl[])
      n198 = Transpose 2D Array(2D array=w329) -> (transposed array=w330:string[][])
      n199 = for {
        tunnel: w321 -> [w418] mode=indexing
        tunnel: [w417] -> w319 mode=indexing
        n200 = Format Into String(w418) -> (resulting string=w417:string)  [unwired: 3 in, 1 out]
      }
      n201 = Build Path(base path=w343, name or relative path=w345) -> (appended path=w337:path)
      n202 = local read "Machine Type"() -> (w311:u8)
      n203 = Build Array(string[] ["FIB FOV (um)", "X center (um)", "Y center (um)", "X size (um)", "Y size (um)", "X resolution ", "Y resolution", "Scan rate (Hz)"] ("Parameter Names"), w319) -> (w318:string[][])
      n204 = case shown="2" w311 {
        frame 0, Default {
        }
        frame 1 {
          w407 = TRUE ("Initialization")
          n205 = local read "COM port"() -> (w401:refnum<visa-resource-name>)
          n206 = call "FIB mode.vi"("Initialization"=w407, "FIB mode"=T8."SEM", "COM port in"=w401) -> ("COM port out"=w402:refnum<visa-resource-name>)  [unwired: 7 in, 1 out]
          n207 = call "Remcon32 command.vi"("SEM command"="edx 0", "COM port in"=w402) -> ("COM port out"=w403:refnum<visa-resource-name>)  [unwired: 6 in, 3 out]
          n208 = call "Remcon32 command.vi"("Close session"=w407, "SEM command"="frez", "COM port in"=w403) -> ()  [unwired: 5 in, 4 out]
        }
        frame 2 {
          n209 = local read "ActiveX Container"() -> (w413:refnum<k7>)
          n210 = invoke class="_EMApi" method="Set"(reference=w413, "lpszParam"="DP_FIB_BLANKER_MODE" ("lpszCommand"), "vValue"=sgl 2.0) -> (reference out=w410:refnum<k7>, error out=w411:errorcluster)  [unwired: 2 in, 3 out]
          n211 = call "SmartSEM Remote API FIB mode.vi"("error in"=w411, "FIB mode"=T9."SEM", "ActiveX Container"=w410) -> ("error out"=w408:errorcluster, "reference out"=w409:refnum<k7>)  [unwired: 7 in]
          n212 = invoke class="_EMApi" method="Execute"(reference=w409, error in=w408, "lpszCommand"="CMD_FREEZE_ALL") -> ()  [unwired: 1 in, 4 out]
        }
      }
      n213 = Build Array (concatenate)(w330, w313, w318, w313, w312) -> (w331:string[][])
      n214 = call-poly <vilib>:"Write To Spreadsheet File.vi"("delimiter (\\t)"="," ("delimiter (\\t)"), "transpose? (no:F)"=TRUE, "2D data"=w331, "file path (dialog if empty)"=w337) -> ()  [unwired: 4 in, 1 out]
    }
    frame #3 {
      n215 = local write "stop"(FALSE ("stop")) -> ()
    }
  }
